vi "Write Analogue.vi"(8 "error in (no error)":errorcluster, 9 "output":bool, 10 "Channel index":i32, 11 "Sim DC Power in":refnum<class "Sim DC Power.lvclass">) -> (0 "error out":errorcluster, 2 "Success?":bool=TRUE, 3 "Sim DC Power out":refnum<class "Sim DC Power.lvclass">)   [LabVIEW 2025, in "Power Supply.lvlib" / "Sim DC Power.lvclass"]
uses:
  Sim DC Power.lvclass
  Sim DC Power.lvclass/Sim DC Power.ctl
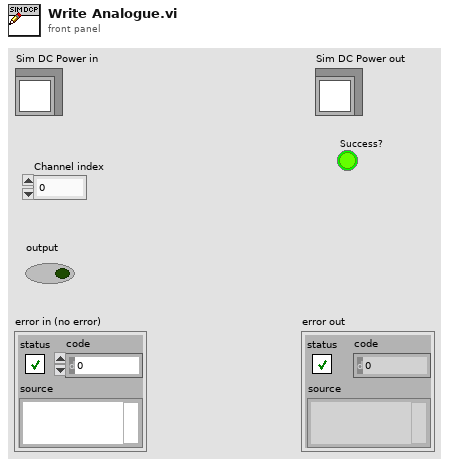
[diagram p1: front panel]
types:
  T1 = typedef "Abstract Engine.lvlibp/Abstract Instrument.lvclass/Channel.ctl" = cluster{"Alias":string, "Type":enum16{"Numeric", "Boolean", "String"}, "Unit":T2, "Upper limit":dbl, "Lower limit":dbl, "Measurement":variant}
  T2 = typedef "Abstract Engine.lvlibp/Abstract Instrument.lvclass/Unit.ctl" = enum16{"---", "V", "A", "Ohm", "Hz", "uF", "degC", "deg"}
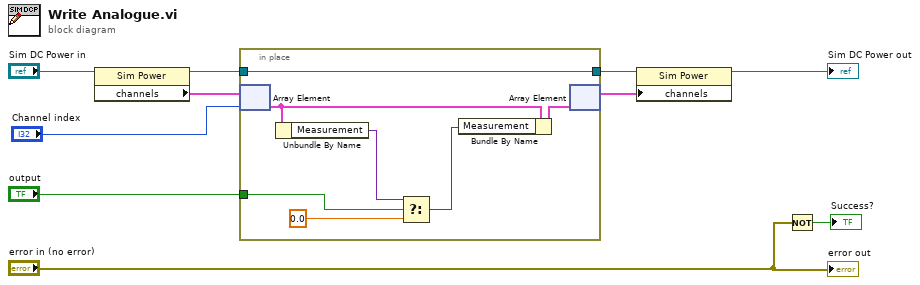
[diagram p0: block diagram]
diagram:
  n1 = property class="Sim Power"(reference="Sim DC Power in") -> (reference out=w6:refnum<class "Sim DC Power.lvclass">, "channels"=w3:T1[])  [unwired: 1 in, 1 out]
  n2 = in-place {
    in-place-border: "output" -> [w16]
    in-place-border: [w15] -> w5
    in-place-border: w6 -> [w15]
    n3 = in-place-array #1(w3, "Channel index") -> (w12:T1)
    n4 = Unbundle By Name(w12) -> ("Measurement"=w11:variant)
    n5 = Select(t=w11, s=w16, f=0.0 ("Voltage")) -> (s? t:f=w13:variant)
    n6 = Bundle By Name(cluster=w12, "Measurement"=w13) -> (w17:T1)
    n7 = in-place-array #1(w17) -> (w1:T1[])  [unwired: 1 out]
  }
  n8 = property class="Sim Power"(reference=w5, "channels"=w1) -> (reference out=→"Sim DC Power out":refnum<class "Sim DC Power.lvclass">)  [unwired: 1 in, 1 out]
  n9 = Not(x="error in (no error)") -> (.not. x?=→"Success?":bool)
  "error out" <- "error in (no error)"
